vi "Load Plugins.vi"(8 "error in (no error)":errorcluster, 11 "Application in":refnum<data-value>) -> (0 "error out":errorcluster, 3 "Application out":refnum<data-value>)   [LabVIEW 2015, in "Application.lvclass"]
uses:
  Application.lvclass
  Plugin.lvclass
  Member Access/Read Path.vi
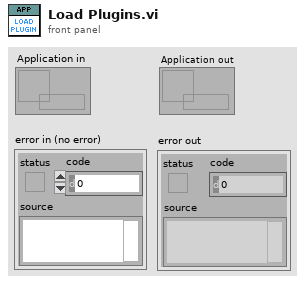
[diagram p1: front panel]
types:
  T1 = typedef "Application Config Typedef.ctl" = cluster{"Auto Load Project":bool, "Project Path":string, "Plugin Folders":string}
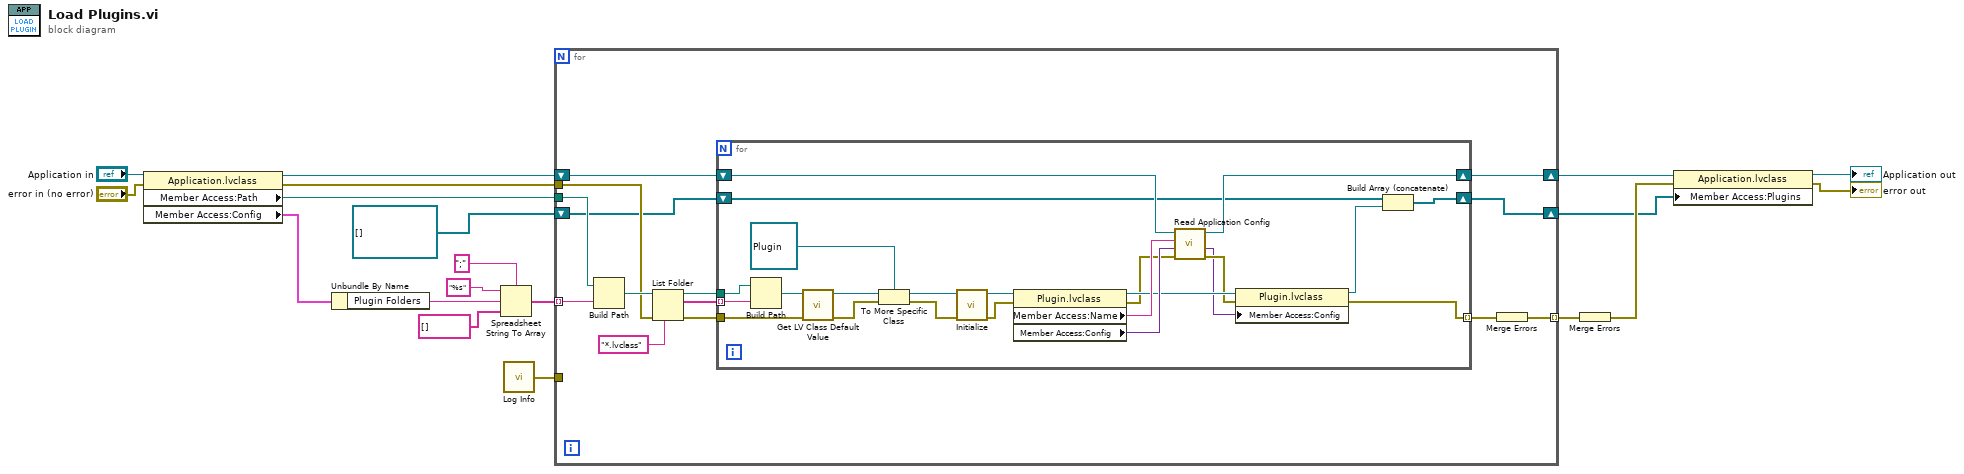
[diagram p0: block diagram]
diagram:
  n1 = property class="Application.lvclass"(reference="Application in", error in="error in (no error)") -> (reference out=w13:refnum<data-value>, error out=w14:errorcluster, "Member Access:Path"=w15:path, "Member Access:Config"=w12:T1)
  n2 = Unbundle By Name(w12) -> ("Plugin Folders"=w8:string)
  n3 = Spreadsheet String To Array(delimiter (Tab)=";", format string="%s", spreadsheet string=w8, array type (2D Dbl)=string[] []) -> (array=w6:string[])
  n4 = call "Log Info.vi"() -> ("error out"=w4:errorcluster)  [unwired: 5 in]
  n5 = for {
    tunnel: w15 -> [w29]
    tunnel: w14 -> [w27]
    shift-right: [w25] -> w7
    shift-left: w13 -> [w26]
    tunnel: w6 -> [w24] mode=indexing
    tunnel: w4 -> [_]
    tunnel: [w22] -> w3 mode=indexing
    shift-right: [w20] -> w1
    shift-left: refnum<class "Plugin.lvclass">[] [] -> [w21]
    n6 = Build Path(base path=w29, name or relative path=w24) -> (appended path=w28:path)
    n7 = List Folder(path=w28, pattern="*.lvclass", error in=w27) -> (path out=w31:path, filenames=w32:string[], error out=w30:errorcluster)  [unwired: 1 in, 1 out]
    n8 = for {
      tunnel: w32 -> [w55] mode=indexing
      tunnel: w31 -> [w56]
      tunnel: w30 -> [w53]
      tunnel: [w37] -> w23 mode=indexing
      shift-right: [w42] -> w25
      shift-left: w26 -> [w43]
      shift-right: [w35] -> w20
      shift-left: w21 -> [w36]
      n9 = Build Path(base path=w56, name or relative path=w55) -> (appended path=w54:path)
      n10 = call <vilib>:"Get LV Class Default Value.vi"("error in (no error)"=w53, "class path"=w54) -> ("error out"=w52:errorcluster, "object"=w51:refnum<class>)  [unwired: 8 in]
      n11 = To More Specific Class(target class=refnum<class "Plugin.lvclass"> refnum ("Plugin.lvclass"), reference=w51, error in=w52) -> (specific class reference=w49:refnum<class "Plugin.lvclass">, error out=w48:errorcluster)
      n12 = call-dynamic "Initialize.vi"("error in (no error)"=w48, "Plugin in"=w49) -> ("error out"=w46:errorcluster, "Plugin out"=w47:refnum<class "Plugin.lvclass">)  [unwired: 8 in]
      n13 = property class="Plugin.lvclass"(reference=w47, error in=w46) -> (reference out=w41:refnum<class "Plugin.lvclass">, error out=w39:errorcluster, "Member Access:Name"=w45:string, "Member Access:Config"=w44:variant)
      n14 = call "Read Application Config.vi"("error in (no error)"=w39, "Config Type In"=w44, "Section"=w45, "Application in"=w43) -> ("error out"=w40:errorcluster, "Config Data out"=w38:variant, "Application out"=w42:refnum<data-value>)  [unwired: 5 in]
      n15 = property class="Plugin.lvclass"(reference=w41, error in=w40, "Member Access:Config"=w38) -> (reference out=w34:refnum<class "Plugin.lvclass">, error out=w37:errorcluster)
      n16 = Build Array (concatenate)(w36, w34) -> (w35:refnum<class "Plugin.lvclass">[])
    }
    n17 = Merge Errors(w23) -> (w22:errorcluster)
  }
  n18 = Merge Errors(w3) -> (w5:errorcluster)
  n19 = property class="Application.lvclass"(reference=w7, error in=w5, "Member Access:Plugins"=w1) -> (reference out=→"Application out":refnum<data-value>, error out=→"error out":errorcluster)
